vi "file to array.vi"() -> ()   [LabVIEW 2020]
panel:
  out "text":string
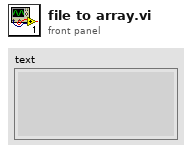
[diagram p1: front panel]
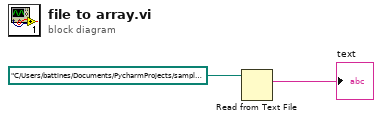
[diagram p0: block diagram]
diagram:
  n1 = Read from Text File(file (use dialog)=path "C:/Users/battines/Documents/PycharmProjects/sample sheet.csv") -> (text=→"text":string)  [unwired: 3 in, 3 out]
